vi "ATC예문.vi"() -> ()   [LabVIEW 2014]
doc: "ATC app"
uses:
  <vilib>/Utility/sysdir.llb/System Directory Type.ctl
panel:
  in  "피드백":bool
  in  "정보1":bool
  in  "도움말":bool
  in  "정규식 5":string
  in  "정규식 4":string
  in  "?":bool
  in  "?":bool
  in  "정규식 3":string
  out "ip address":string="ip address"
  in  "탭":T1(tab)
  in  "메모":string="필요한 메모를 할수 있습니다. "
  in  "SID&RadarVector. 2":string="SID&RadarVector. "
  in  "인사말":string="인사말"
  in  "CD관제기관":string="관제기관"
  in  "콜사인":string="콜사인\n콜사인\n콜사인"
  in  "도착공항":string="도착공항"
  in  "SID&RadarVector":string="SID&RadarVector"
  in  "비행고도":string="비행고도"
  in  "인사말2":string="인사말"
  in  "콜사인2":string="콜사인"
  in  "콜사인3":string="콜사인"
  in  "콜사인4":string="콜사인"
  in  "콜사인5":string="콜사인"
  in  "콜사인6":string="콜사인"
  in  "도착공항2":string="도착공항"
  in  "제한고도":string="제한고도"
  in  "비행고도2":string="비행고도"
  in  "D접속주파수":string="접속주파수"
  in  "스콱번호":string="스콱번호"
  in  "도착공항3":string="도착공항"
  in  "SID&RadarVector. 3":string="SID&RadarVector. "
  in  "제한고도2":string="제한고도"
  in  "비행고도3":string="비행고도"
  in  "D접속주파수2":string="접속주파수"
  in  "스콱번호2":string="스쾃번호"
  in  "콜사인7":string="콜사인"
  in  "콜사인8":string="콜사인"
  in  "G관제기관":string="관제기관"
  in  "G접속주파수2":string="접속주파수"
  in  "G관제기관2":string="관제기관"
  in  "G접속주파수":string="접속주파수"
  in  "콜사인9":string="콜사인"
  in  "유도로 2":string="유도로"
  in  "유도로":string="유도로"
  in  "방향 2":string="방향"
  in  "방향":string="방향"
  in  "메모2":string="필요한 메모를 할수 있습니다. "
  in  "T관제기관2":string="관제기관"
  in  "콜사인24":string="콜사인"
  in  "T접속주파수2":string="접속주파수"
  in  "T접속주파수":string="접속주파수"
  in  "T관제기관":string="관제기관"
  in  "콜사인23":string="콜사인"
  in  "활주로9":string="활주로"
  in  "G관제기관4":string="관제기관"
  in  "콜사인22":string="콜사인"
  in  "콜사인21":string="콜사인"
  in  "콜사인20":string="콜사인"
  in  "콜사인19":string="콜사인"
  in  "활주로8":string="활주로"
  in  "활주로7":string="활주로"
  in  "콜사인17":string="콜사인"
  in  "활주로6":string="활주로"
  in  "콜사인18":string="콜사인"
  in  "활주로5":string="활주로"
  in  "콜사인16":string="콜사인"
  in  "활주로4":string="활주로"
  in  "콜사인15":string="콜사인"
  in  "활주로3":string="활주로"
  in  "콜사인14":string="콜사인"
  in  "콜사인13":string="콜사인"
  in  "현재기압2":string="현재기압"
  in  "출발공항":string="출발공항"
  in  "활주로2":string="활주로"
  in  "현재기압":string="현재기압"
  in  "출발공항2":string="출발공항"
  in  "활주로1":string="활주로"
  in  "콜사인12":string="콜사인"
  in  "콜사인11":string="콜사인"
  in  "G관제기관3":string="관제기관"
  in  "인사3":string="인사"
  in  "콜사인34 2":string="콜사인"
  in  "D관제기관2":string="관제기관"
  in  "D관제기관":string="관제기관"
  in  "T관제기관3":string="관제기관"
  in  "메모3":string="필요한 메모를 할수 있습니다. "
  in  "인사4":string="인사"
  in  "콜사인25":string="콜사인"
  in  "활주로10":string="활주로"
  in  "콜사인26":string="콜사인"
  in  "바람방향":string="바람방향"
  in  "풍속":string="풍속"
  in  "콜사인28":string="콜사인"
  in  "활주로13":string="활주로"
  in  "콜사인29":string="콜사인"
  in  "활주로12":string="활주로"
  in  "콜사인30":string="콜사인"
  in  "활주로14":string="활주로"
  in  "콜사인31":string="콜사인"
  in  "활주로15":string="활주로"
  in  "T관제기관4":string="관제기관"
  in  "콜사인32":string="콜사인"
  in  "현재고도":string="현재고도"
  in  "허가고도":string="허가고도"
  in  "콜사인33":string="콜사인"
  in  "접속주파수":string="접속주파수"
  in  "콜사인34":string="콜사인"
  in  "접속주파수2":string="접속주파수"
  in  "순항고도or이니셜고도":string="순항고도or이니셜고도"
  in  "D관제기관5":string="관제기관"
  in  "메모 4":string="필요한 메모를 할수 있습니다. "
  in  "인사5":string="인사"
  in  "D관제기관3":string="관제기관"
  in  "콜사인35":string="콜사인"
  in  "현재고도A":string="현재고도"
  in  "콜사인36":string="콜사인"
  in  "D관제기관4":string="관제기관"
  in  "허가고도4":string="허가고도"
  in  "허가고도5":string="허가고도"
  in  "콜사인37":string="콜사인"
  in  "콜사인38":string="콜사인"
  in  "허가고도6":string="허가고도"
  in  "허가고도7":string="허가고도"
  in  "콜사인39":string="콜사인"
  in  "콜사인40":string="콜사인"
  in  "C관제기관":string="관제기관"
  in  "A접속주파수":string="접속주파수"
  in  "C관제기관2":string="관제기관"
  in  "A접속주파수2":string="접속주파수"
  in  "콜사인41":string="콜사인"
  in  "콜사인38 2":string="콜사인"
  in  "D관제기관6":string="관제기관"
  in  "허가고도6 2":string="허가고도"
  in  "허가고도6 3":string="허가고도"
  in  "콜사인39 2":string="콜사인"
  in  "메모5":string="필요한 메모를 할수 있습니다. "
  in  "인사말 2":string="인사말"
  in  "허가고도 2":string="허가고도"
  in  "지점":string="지점"
  in  "허가고도7 2":string="허가고도"
  in  "콜사인38 3":string="콜사인"
  in  "콜사인39 3":string="콜사인"
  in  "허가고도7 3":string="허가고도"
  in  "지점 2":string="지점"
  in  "메모6":string="필요한 메모를 할수 있습니다. "
  in  "A관제기관3":string="관제기관"
  in  "콜사인46":string="콜사인"
  in  "날시정보":string="날시정보"
  in  "고도":string="고도"
  in  "콜사인47":string="콜사인"
  in  "A관제기관4":string="관제기관"
  in  "L활주로":string="활주로"
  in  "도착공항4":string="도착공항"
  in  "현재기압":string="현재기압"
  in  "콜사인48":string="콜사인"
  in  "A관제기관5":string="관제기관"
  in  "L활주로":string="활주로"
  in  "도착공항5":string="도착공항"
  in  "현재기압":string="현재기압"
  in  "콜사인49":string="콜사인"
  in  "고도":string="고도"
  in  "콜사인50":string="콜사인"
  in  "고도":string="고도"
  in  "콜사인51":string="콜사인"
  in  "고도":string="고도"
  in  "고도":string="고도"
  in  "콜사인52":string="콜사인"
  in  "콜사인53":string="콜사인"
  in  "A관제기관":string="관제기관"
  in  "풍속":string="풍속"
  in  "바람방향":string="바람방향"
  in  "L활주로3":string="활주로"
  in  "콜사인54":string="콜사인"
  in  "L활주로":string="활주로"
  in  "콜사인55":string="콜사인"
  in  "A관제기관2":string="관제기관"
  in  "L활주로":string="활주로"
  in  "ILS":string="주파수(ils)"
  in  "콜사인56":string="콜사인"
  in  "L활주로6":string="활주로"
  in  "ILS2":string="주파수(ils)"
  in  "콜사인57":string="콜사인"
  in  "T관제기관":string="관제기관"
  in  "T접속주파수":string="접속주파수"
  in  "콜사인58":string="콜사인"
  in  "콜사인59":string="콜사인"
  in  "관제기관":string="관제기관"
  in  "T접속주파수":string="접속주파수"
  in  "메모7":string="필요한 메모를 할수 있습니다. "
  in  "바람방향":string="바람방향"
  in  "관제기관":string="관제기관"
  in  "콜사인60":string="콜사인"
  in  "L활주로7":string="활주로"
  in  "콜사인61":string="콜사인"
  in  "풍속":string="풍속"
  in  "콜사인62":string="콜사인"
  in  "L활주로":string="활주로"
  in  "L활주로":string="활주로"
  in  "관제기관":string="관제기관"
  in  "콜사인63":string="콜사인"
  in  "관제기관3":string="관제기관"
  in  "콜사인64":string="콜사인"
  in  "L활주로":string="활주로"
  in  "G관제기관":string="관제기관"
  in  "G접속주파수":string="접속주파수"
  in  "콜사인65":string="콜사인"
  in  "관제기관":string="관제기관"
  in  "G접속주파수":string="접속주파수"
  in  "콜사인70":string="콜사인"
  in  "C활주로3":string="활주로"
  in  "C활주로2":string="활주로"
  in  "관제기관3 2":string="관제기관"
  in  "C활주로":string="활주로"
  in  "콜사인69":string="콜사인"
  in  "관제기관2":string="관제기관"
  in  "메모8":string="필요한 메모를 할수 있습니다. "
  in  "관제기관":string="관제기관"
  in  "콜사인66":string="콜사인"
  in  "콜사인67":string="콜사인"
  in  "게이트번호":string="게이트번호"
  in  "THEN":string="then"
  in  "콜사인68":string="콜사인"
  in  "게이트번호2":string="게이트번호"
  in  "THEN2":string="then"
  in  "콜사인10":string="콜사인"
  in  "관제기관4":string="관제기관"
  in  "콜사인71":string="콜사인"
  in  "콜사인72":string="콜사인"
  # "ver.3.0.0.55"
  # "~"
  # "Good"
  # "Clearance Delivery"
  # "Pilot"
  # "at FL"
  # "Request IFR Clearance to"
  # "Airport via"
  # "~"
  # "Good"
  # "Controller"
  # ",  Clearance  Delivery, standby."
  # "Pilot"
  # "Stand by,"
  # "Controller"
  # "Delivery 또는 Delivery, Are you ready to copy?"
  # "Pilot"
  # "Go Ahead 또는 Ready to copy"
  # "Airport via"
  # ", Cleared to"
  # "Controller"
  # "ft expect FL"
  # "then as filed. Climb and Maintain"
  # "Departure Frequency"
  # "Read back."
  # "Squawk"
  # "Pilot"
  # "Airport via"
  # "Cleared to"
  # ","
  # "then as filed."
  # "Climb and Maintain"
  # "ft expect FL"
  # "Departure Frequency"
  # "and  Squawk"
  # "Controller"
  # ", Read back is corrent contact"
  # "Ground"
  # "bye bye~."
  # "Pilot"
  # "Roger, contact"
  # ", bye bye~"
  # "Pilot"
  # "Good"
  # "~"
  # "ready for push back and Engine Start."
  # ","
  # ", Rwy"
  # "Push Back and Engine Start Approved, heading to"
  # "Controller"
  # ","
  # "QNH"
  # "Read Back."
  # "Pilot"
  # "Roger\nPush Back and Engine Start Approved, heading to"
  # ", Rwy"
  # "QNH"
  # "Ready for taxi to the Rwy"
  # ","
  # "Pilot"
  # "- Push back 완료 후 -"
  # ", Ready for Taxi to Rwy"
  # "Controller"
  # ", taxi to"
  # "via taxiway"
  # ", Roger"
  # "Pilot"
  # "via taxiway"
  # "Taxi to"
  # "- 활주로를 건널 상황일 때 -"
  # "Pilot"
  # "Request Cross Rwy"
  # "Controller"
  # ", cleared Cross Rwy"
  # "Pilot"
  # "cleared Cross Rwy"
  # "Controller"
  # "Squawk Mode C."
  # "Pilot"
  # ", Roger squawk mode 'C'"
  # "------------------------ 홀딩 포인트 도착 후 ----------------------------------"
  # "Pilot"
  # "hold short of Rwy"
  # ","
  # "Controller"
  # "Roger,"
  # "contact"
  # "Tower"
  # "bye bye~"
  # "Pilot"
  # "Contact"
  # "Pilot"
  # "Good"
  # "~"
  # ",  hold short Rwy"
  # ", Ready for Departure"
  # "(곧바로 이륙허가)"
  # "Controller"
  # ", wind"
  # "knot, cleared for take off."
  # "at"
  # "(활주로 정렬대기)"
  # "Controller"
  # "Line up and wait Rwy"
  # "Pilot"
  # "Line up and wait Rwy"
  # "Roger,"
  # "(홀딩 포인트에서 대기)"
  # "Controller"
  # ", Hold short rwy"
  # ","
  # "Pilot"
  # "Hold short of Rwy"
  # "Roger,"
  # "- 이 륙 후 -"
  # "Pilot"
  # "ft."
  # "Airborn Passing"
  # "ft, Climbing"
  # ","
  # "Controller"
  # ", contact"
  # "Departure,"
  # "bye bye~"
  # "Pilot"
  # ", Roger"
  # "Contact"
  # "Departure,"
  # "bye bye~"
  # "Good"
  # "~"
  # "Pilot"
  # "Passing"
  # "expect"
  # "with (SID)."
  # ","
  # ","
  # "Controller"
  # "Departure, Radar Contact, Climb via (SID) to"
  # ","
  # "."
  # "Pilot"
  # "Roger, Climb via"
  # ","
  # "-고도제한 해제시-"
  # "Controller"
  # "Departure, Radar Contact, Climb via (SID) to"
  # ", Cancel Level Restrictions."
  # "Pilot"
  # "Roger, Climb via (SID) to"
  # ", Cancel Level Restrictions,"
  # "-속도제한 해제시-"
  # "Controller"
  # "Departure, Radar Contact, Climb via (SID) to"
  # ", Cancel Speed Restrictions."
  # "Pilot"
  # "Roger, Climb via (SID) to"
  # ", Cancel Speed Restrictions,"
  # "Controller"
  # "Control,"
  # ", bye bye."
  # ", You are leaving my airspace, Contact"
  # "Pilot"
  # "Contact"
  # "G'day"
  # "Control,"
  # ","
  # "Pilot"
  # "Good"
  # "Decend and maintain FL"
  # "with (SID)."
  # "-하강 발부-"
  # "Controller"
  # "by"
  # ", Descend and Maintain"
  # "Pilot"
  # "Descend and Maintain"
  # "by"
  # "Pilot"
  # ","
  # "FL"
  # "with information"
  # ","
  # ", Expect vector to ILS Rwy"
  # "approach"
  # "Controller"
  # "QNH"
  # "Roger,"
  # "Pilot"
  # ", Expect vector to ILS Rwy"
  # "final approach"
  # "QNH"
  # "Controller"
  # ", Decend and maintain FL"
  # "Pilot"
  # "Decend and maintain FL"
  # "Roger,"
  # "Controller"
  # ", Decend and maintain"
  # "ft"
  # "Pilot"
  # "Roger"
  # "Decend and maintain"
  # "ft"
  # "Controller"
  # ","
  # "for landing"
  # "wind"
  # "knots active Rwy"
  # "at"
  # "Pilot"
  # "Roger,"
  # "Rwy"
  # "for landing"
  # "Controller"
  # ","
  # "approach use Rwy"
  # "ILS"
  # "Roger,"
  # "Pilot"
  # "Use Rwy"
  # "ILS"
  # "- 정 렬 후 -"
  # "Pilot"
  # "Approach,"
  # ", Established on Localizer."
  # "Controller"
  # "Tower,"
  # "Good day,"
  # "Roger, Contact"
  # "Pilot"
  # "Contact"
  # "Tower"
  # "Good day,"
  # "Pilot"
  # ","
  # "Inbound Approaching Rwy"
  # "Controller"
  # ", Wind"
  # "at"
  # "knots Rwy"
  # ", Cleared to land"
  # "Pilot"
  # "Rwy"
  # "Cleared to land"
  # "Pilot"
  # ","
  # "- 착 륙 후 -"
  # ","
  # "Pilot"
  # "Touch down with Rwy"
  # "Controller"
  # "Roger, change squawk mode Standby and contact"
  # "bye bye~"
  # "ground"
  # "Pilot"
  # ", Roger"
  # "bye bye~"
  # "Change squawk mode standby and contact"
  # "- 활주로를 건널 상황일 때 -"
  # "Pilot"
  # ","
  # "Request Cross Rwy"
  # "Controller"
  # ", Cross Rwy"
  # "approved."
  # "Pilot"
  # "Cross Rwy"
  # "approved"
  # ","
  # "Pilot"
  # "Ready to taxi to the Gate"
  # "Controller"
  # ", taxi to the gate"
  # "via taxi way"
  # "Roger,"
  # "Pilot"
  # "taxi to the gate"
  # "via taxi way"
  # "- 게이트 도착 후 -"
  # "Pilot"
  # "at Gate and Engine Shut down."
  # "Thank you for your ATC service."
  # "Controller"
  # ", at the gate and Engine Shut down, Thank you ~~"
  # "Pilot"
  # "Have a nice day,"
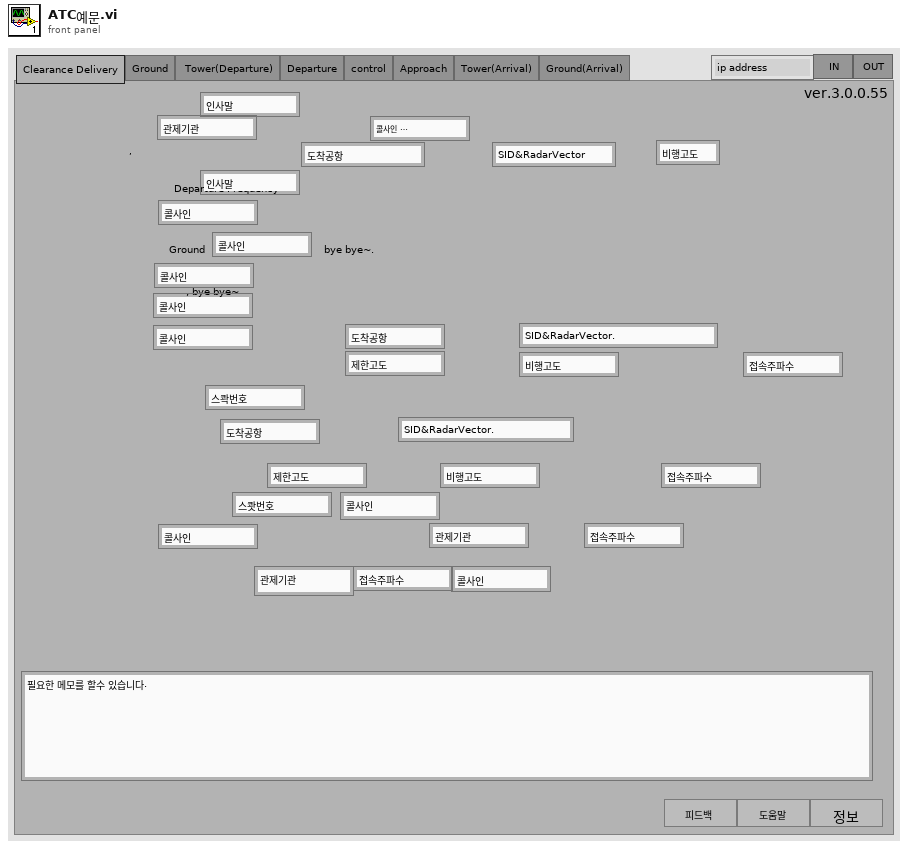
[diagram p1: front panel]
types:
  T1 = enum32{"Clearance Delivery", "Ground", " Tower(Departure)", "Departure", "control", "Approach", "Tower(Arrival)", "Ground(Arrival)"}
  T2 = enum16{"open", "replace", "create", "open or create", "replace or create", "replace or create with confirmation"}
  T3 = typedef "System Directory Type.ctl" = i32
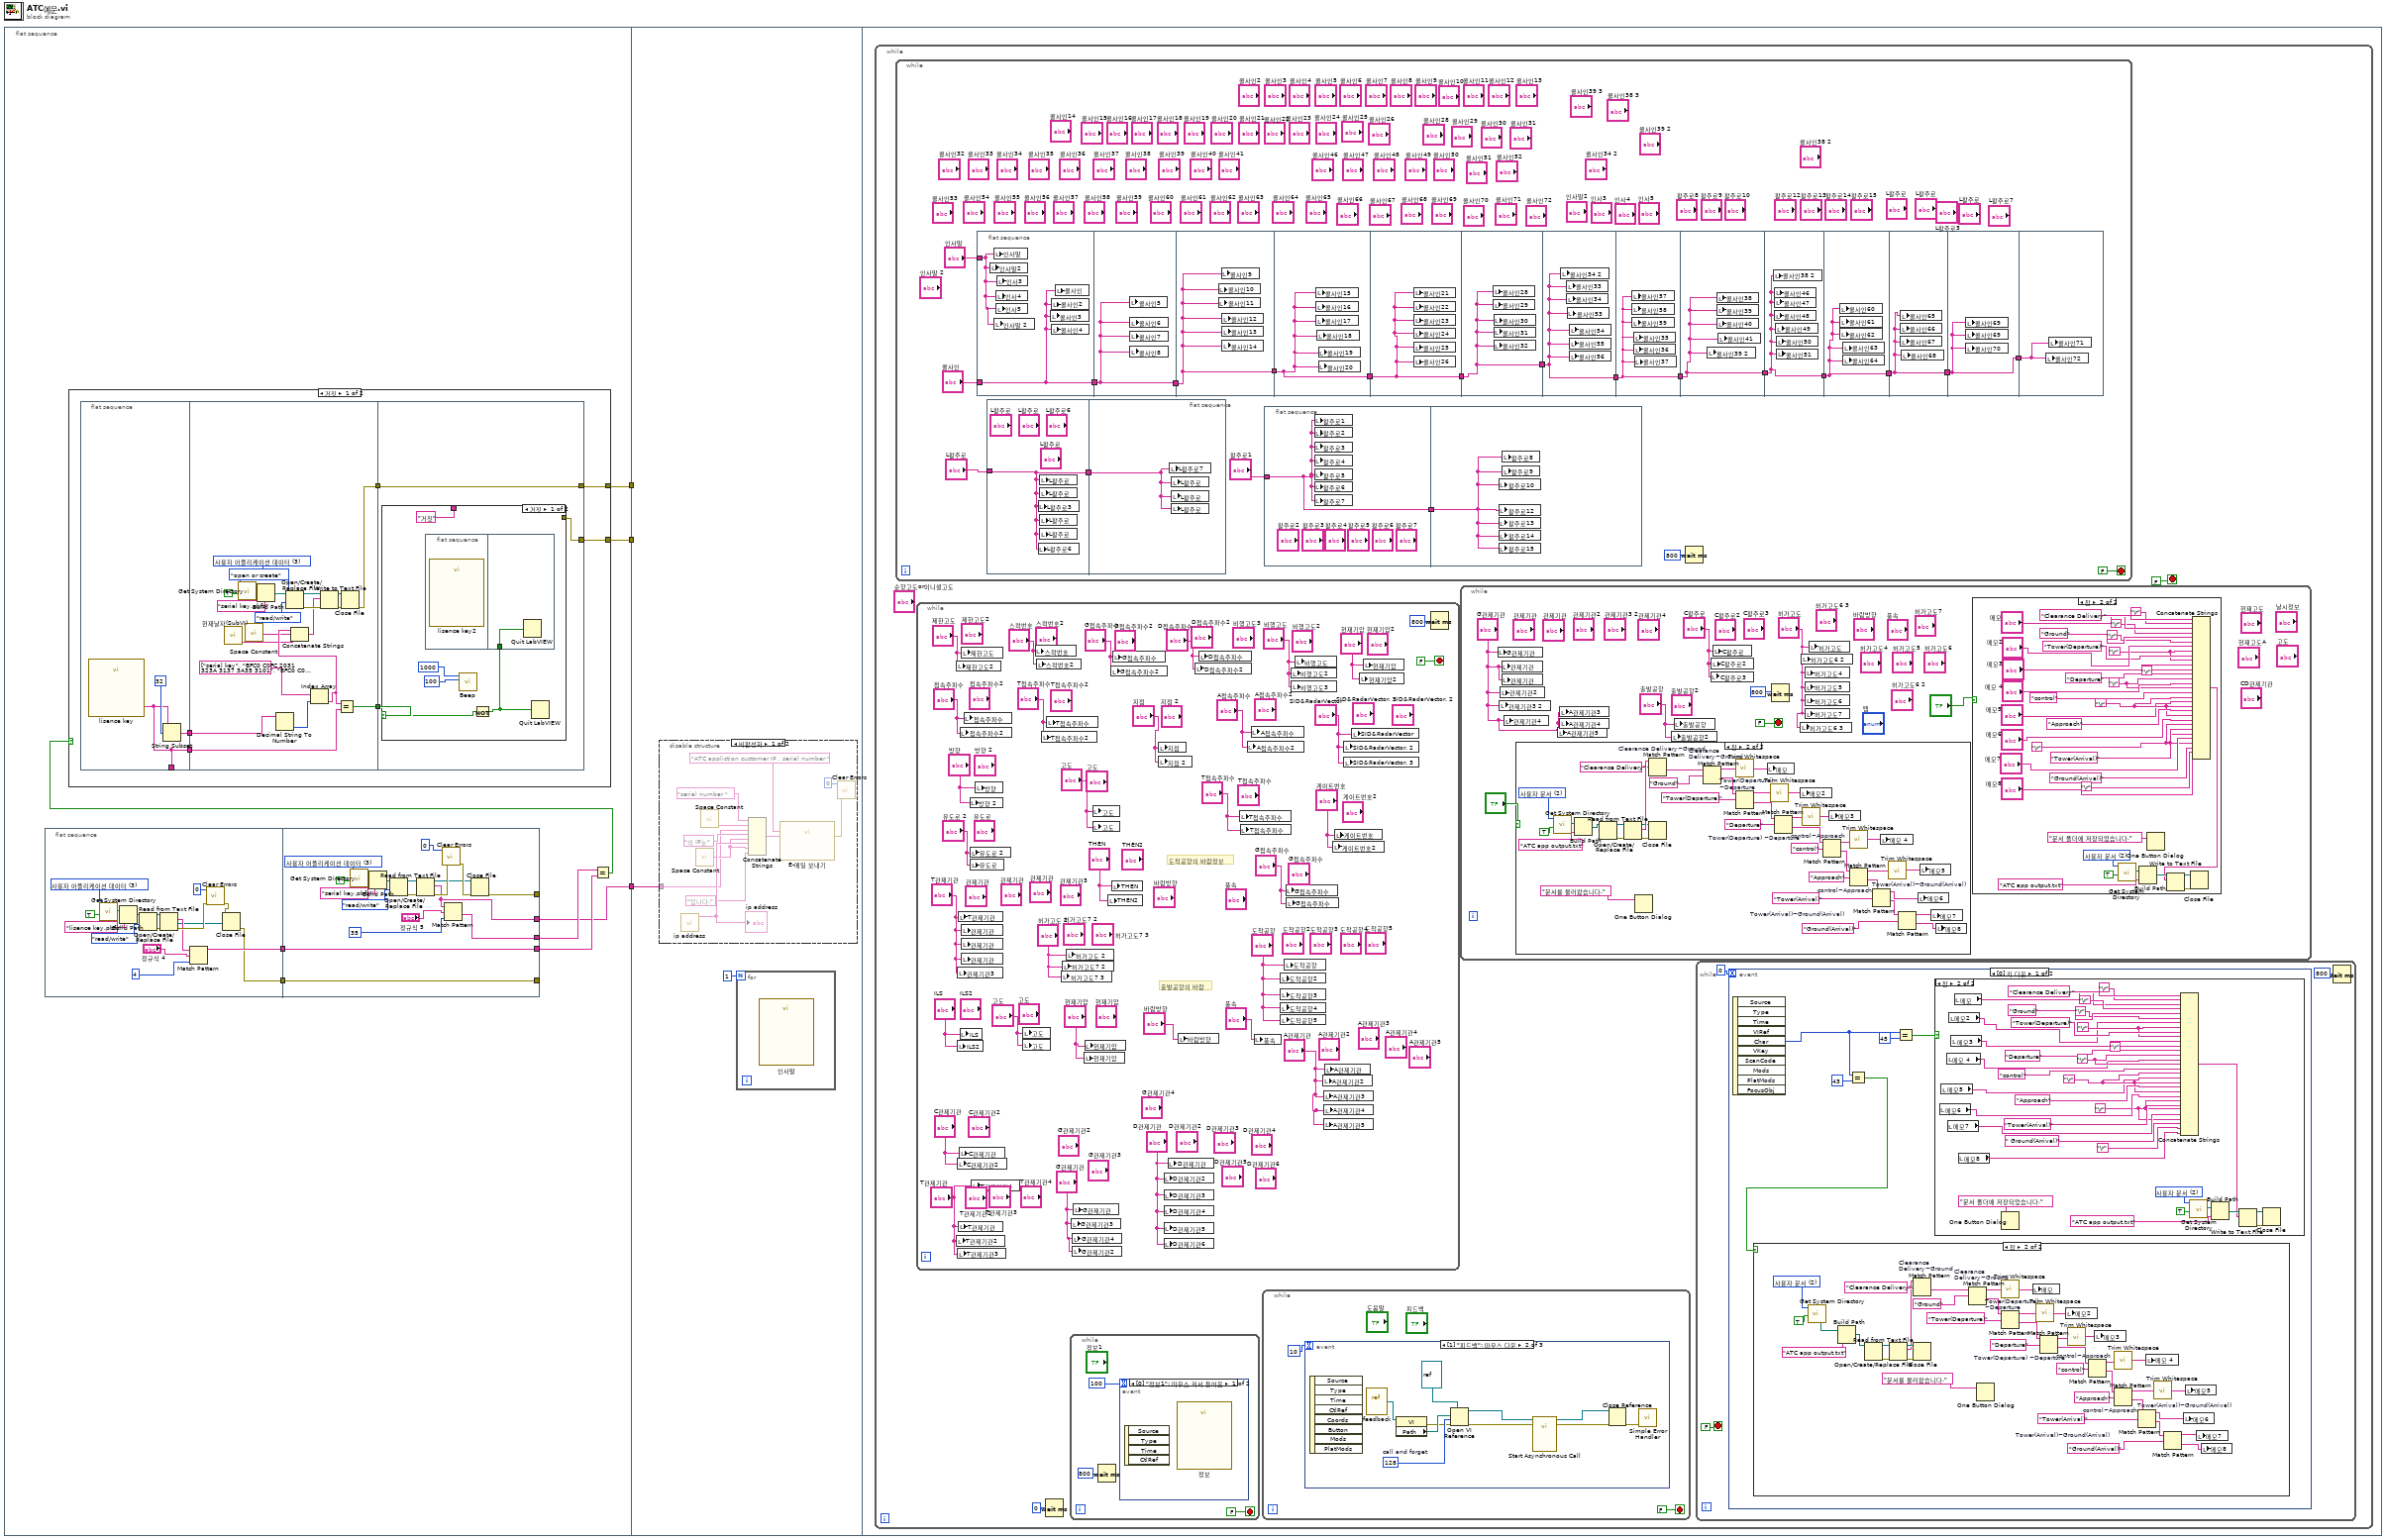
[diagram p0: block diagram]
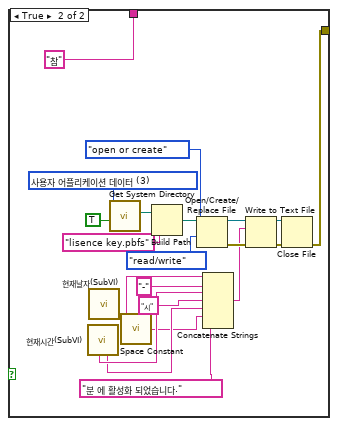
[diagram p2: hidden frame]
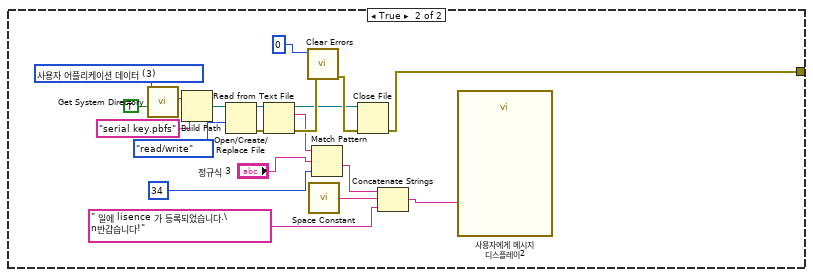
[diagram p3: hidden frame]
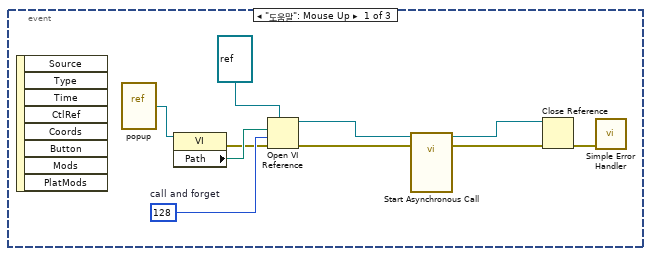
[diagram p5: hidden frame]
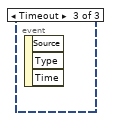
[diagram p6: hidden frame]
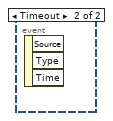
[diagram p9: hidden frame]
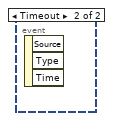
[diagram p10: hidden frame]
diagram:
  n1 = flat-sequence {
    tunnel: [w4] -> w3
    tunnel: [w11] -> w2
    tunnel: [w10] -> w1
    tunnel: w3 -> [w128]
    tunnel: w2 -> [_]
    tunnel: w1 -> [_]
    frame #0 {
      n2 = flat-sequence {
        tunnel: [w13] -> w9
        tunnel: [w12] -> w8
        tunnel: [w35] -> w6
        tunnel: w9 -> [w35]
        tunnel: [w33] -> w7
        tunnel: [w29] -> w4
        tunnel: [w31] -> _
        tunnel: w8 -> [w31]
        tunnel: [w30] -> _
        frame #0 {
          w18 = T3 3 items=["사용자 홈"=0, "사용자 데스크탑"=1, "사용자 문서"=2, "사용자 어플리케이션 데이터"=3, "사용자 환경"=4, "사용자 임시"=5, "퍼블릭 문서"=6, "퍼블릭 어플리케이션 데이터"=7, "퍼블릭 환경"=8, "퍼블릭 캐시"=13, "시스템 코어 라이브러리"=9, "시스템 설치된 라이브러리"=10, "어플리케이션 파일"=11, "부팅 볼륨 루트"=12] ("system directory type")
          n3 = call <vilib>:"Get System Directory.vi"("create directory if not found? (F)"=TRUE, "system directory type"=w18) -> ("system directory"=w17:path)  [unwired: 9 in]
          n4 = Build Path(base path=w17, name or relative path="lisence key.pbfs" ("이름 또는 상대 경로")) -> (appended path=w16:path)
          n5 = Open/Create/Replace File(file path (use dialog)=w16, access (0:read/write)=enum16{"read/write", "read-only", "write-only"}."read/write" ("접근(0:읽기/쓰기)")) -> (refnum out=w22:refnum<file>, error out=w21:errorcluster)  [unwired: 4 in, 1 out]
          n6 = Read from Text File(file (use dialog)=w22, error in=w21) -> (refnum out=w23:refnum<file>, text=w24:string, error out=w26:errorcluster)  [unwired: 2 in, 1 out]
          n7 = Match Pattern(string=w24, regular expression="정규식 4", offset (0)=4 ("오프셋(0) 2")) -> (before substring=w13:string)  [unwired: 3 out]
          n8 = call <vilib>:"Clear Errors.vi"("error in (no error)"=w26, "specific error code to clear (0: all)"=0) -> ("error out"=w27:errorcluster)  [unwired: 4 in, 1 out]
          n9 = Close File(refnum=w23, error in=w27) -> (error out=w12:errorcluster)  [unwired: 1 out]
        }
        frame #1 {
          w41 = T3 3 items=["사용자 홈"=0, "사용자 데스크탑"=1, "사용자 문서"=2, "사용자 어플리케이션 데이터"=3, "사용자 환경"=4, "사용자 임시"=5, "퍼블릭 문서"=6, "퍼블릭 어플리케이션 데이터"=7, "퍼블릭 환경"=8, "퍼블릭 캐시"=13, "시스템 코어 라이브러리"=9, "시스템 설치된 라이브러리"=10, "어플리케이션 파일"=11, "부팅 볼륨 루트"=12] ("system directory type")
          n10 = call <vilib>:"Get System Directory.vi"("create directory if not found? (F)"=TRUE, "system directory type"=w41) -> ("system directory"=w42:path)  [unwired: 9 in]
          n11 = Build Path(base path=w42, name or relative path="serial key.pbfs" ("이름 또는 상대 경로")) -> (appended path=w43:path)
          n12 = Open/Create/Replace File(file path (use dialog)=w43, access (0:read/write)=enum16{"read/write", "read-only", "write-only"}."read/write" ("접근(0:읽기/쓰기)")) -> (refnum out=w37:refnum<file>, error out=w38:errorcluster)  [unwired: 4 in, 1 out]
          n13 = Read from Text File(file (use dialog)=w37, error in=w38) -> (refnum out=w36:refnum<file>, text=w29:string, error out=w45:errorcluster)  [unwired: 2 in, 1 out]
          n14 = call <vilib>:"Clear Errors.vi"("error in (no error)"=w45, "specific error code to clear (0: all)"=0) -> ("error out"=w46:errorcluster)  [unwired: 4 in, 1 out]
          n15 = Match Pattern(string=w29, regular expression="정규식 5", offset (0)=35 ("오프셋(0)")) -> (after substring=w33:string)  [unwired: 3 out]
          n16 = Close File(refnum=w36, error in=w46) -> (error out=w30:errorcluster)  [unwired: 1 out]
        }
      }
      n17 = Equal?(x=w7, y=w6) -> (x = y?=w5:bool)
      n18 = case shown="거짓" w5 {
        tunnel: [w49 w108] -> w10
        tunnel: [w48 _] -> w11
        frame False {
          n19 = flat-sequence {
            tunnel: [w55] -> w53
            tunnel: [w54] -> w52
            tunnel: [w54] -> _
            tunnel: w53 -> [w77]
            tunnel: [w74] -> w51
            tunnel: w52 -> [w75]
            tunnel: [w58] -> w50
            tunnel: w51 -> [w80]
            tunnel: [w79] -> w49
            tunnel: w50 -> [w78]
            tunnel: [w78] -> w48
            frame #0 {
              n20 = call "lisence key"() -> ("lisence key"=w54:string)  [unwired: 17 in, 2 out]
              n21 = String Subset(string=w54, offset (0)=32 ("오프셋(0)")) -> (substring=w55:string)  [unwired: 1 in]
            }
            frame #1 {
              w67 = T3 3 items=["사용자 홈"=0, "사용자 데스크탑"=1, "사용자 문서"=2, "사용자 어플리케이션 데이터"=3, "사용자 환경"=4, "사용자 임시"=5, "퍼블릭 문서"=6, "퍼블릭 어플리케이션 데이터"=7, "퍼블릭 환경"=8, "퍼블릭 캐시"=13, "시스템 코어 라이브러리"=9, "시스템 설치된 라이브러리"=10, "어플리케이션 파일"=11, "부팅 볼륨 루트"=12] ("system directory type")
              n22 = call "현재날자(SubVI).vi"() -> ("월,일 을 문자열로"=w62:string)  [unwired: 5 in, 6 out]
              n23 = call <vilib>:"Get System Directory.vi"("create directory if not found? (F)"=TRUE, "system directory type"=w67) -> ("system directory"=w66:path)  [unwired: 9 in]
              n24 = call <vilib>:"Space Constant.vi"() -> ("String"=w61:string)
              n25 = Build Path(base path=w66, name or relative path="serial key.pbfs" ("이름 또는 상대 경로")) -> (appended path=w65:path)
              n26 = Decimal String To Number(string=w77) -> (number=w76:i32)  [unwired: 2 in, 1 out]
              n27 = Open/Create/Replace File(file path (use dialog)=w65, operation (0:open)=T2."open or create" ("동작(0:open)"), access (0:read/write)=enum16{"read/write", "read-only", "write-only"}."read/write" ("접근(0:읽기/쓰기)")) -> (refnum out=w73:refnum<file>, error out=w72:errorcluster)  [unwired: 3 in, 1 out]
              n28 = Index Array(array=string[] ["serial key", "BFC0 C0FC 2031 323A 3137 3A35 3101", "BFC0 C0FC 2031 323A 3138 3A30 3902", "BFC0 C0FC 2031 323A 3139 3A30 3903", "BFC0 C0FC 2031 323A 3230 3A30 3904", "BFC0 C0FC 2031 323A 3231 3A30 3905", "BFC0 C0FC 2031 323A 3232 3A30 3906", "BFC0 C0FC 2031 323A 3233 3A30 3907", "BFC0 C0FC 2031 323A 3234 3A30 3908", "BFC0 C0FC 2031 323A 3235 3A30 3909", "BFC0 C0FC 2031 323A 3236 3A30 3910", "BFC0 C0FC 2031 323A 3237 3A30 3911", "BFC0 C0FC 2031 323A 3238 3A30 3912", "BFC0 C0FC 2031 323A 3239 3A30 3913", "BFC0 C0FC 2031 323A 3036 3A33 3214", "BFC0 C0FC 2031 323A 3037 3A33 3215", "BFC0 C0FC 2031 323A 3038 3A33 3216", "BFC0 C0FC 2031 323A 3038 3A33 3217", "BFC0 C0FC 2031 323A 3039 3A33 3218", "BFC0 C0FC 2031 323A 3039 3A35 3019", "BFC0 C0FC 2031 323A 3130 3A35 3020", "BFC0 C0FC 2031 323A 3131 3A35 3121", "BFC0 C8C4 2031 313A 3536 3A33 3222", "BFC0 C8C4 2031 313A 3537 3A33 3223", "BFC0 C8C4 2031 313A 3538 3A33 3224", "BFC0 C8C4 2031 313A 3539 3A33 3225", "BFC0 C0FC 2031 323A 3030 3A33 3226", "BFC0 C0FC 2031 323A 3031 3A33 3227", "BFC0 C0FC 2031 323A 3032 3A33 3228", "BFC0 C0FC 2031 323A 3033 3A33 3229", "BFC0 C0FC 2031 323A 3034 3A33 3230", "BFC0 C0FC 2031 323A 3035 3A33 3231", "BFC0 C0FC 2031 323A 3036 3A33 3232", "BFC0 C0FC 2031 323A 3037 3A33 3233", "BFC0 C0FC 2031 323A 3038 3A33 3234", "BFC0 C0FC 2033 3A34 373A 3031 0035 ", "BFC0 C0FC 2033 3A34 383A 3234 0036", "BFC0 C0FC 2033 3A34 393A 3132 0037", "BFC0 C0FC 2033 3A35 303A 3534 0038", "BFC0 C0FC 2033 3A35 313A 3231 0039 ", "BFC0 C0FC 2033 3A35 323A 3333 0040 ", "BFC0 C0FC 2033 3A35 333A 3030 0041", "BFC0 C0FC 2033 3A35 343A 3432 0042", "BFC0 C0FC 2033 3A35 353A 3431 0043", "BFC0 C0FC 2033 3A35 363A 3131 0044", "BFC0 C0FC 2033 3A35 373A 3239 0045", "BFC0 C0FC 2033 3A35 383A 3539 0046", "BFC0 C0FC 2033 3A35 393A 3533 0047", "BFC0 C0FC 2034 3A30 303A 3430 0048 "] ("출력 배열"), index=w76) -> (element=w63:string)
              n29 = Concatenate Strings(w63, w61, w62) -> (w64:string)
              n30 = Write to Text File(file (use dialog)=w73, text=w64, error in=w72) -> (refnum out=w70:refnum<file>, error out=w71:errorcluster)  [unwired: 1 in, 1 out]
              n31 = Equal?(x=w63, y=w75) -> (x = y?=w74:bool)
              n32 = Close File(refnum=w70, error in=w71) -> (error out=w58:errorcluster)  [unwired: 1 out]
            }
            frame #2 {
              n33 = case shown="거짓" w80 {
                selector: w80 -> [w83 _]
                tunnel: ["거짓" "참"] -> _
                tunnel: [_ w87] -> w79
                frame False {
                  n34 = flat-sequence {
                    tunnel: w84 -> [w86]
                    frame #0 {
                      n35 = call "lisence key2"() -> ()  [unwired: 10 in, 2 out]
                    }
                    frame #1 {
                      n36 = Quit LabVIEW(quit? (T)=w86) -> ()
                    }
                  }
                  n37 = call <vilib>:"Beep.vi"("duration (msec)"=u32 100, "frequency (Hz)"=u32 1000) -> ()  [unwired: 10 in]
                  n38 = Not(x=w83) -> (.not. x?=w84:bool)
                  n39 = Quit LabVIEW(quit? (T)=w84) -> ()
                }
                frame True {
                  w103 = T3 3 items=["사용자 홈"=0, "사용자 데스크탑"=1, "사용자 문서"=2, "사용자 어플리케이션 데이터"=3, "사용자 환경"=4, "사용자 임시"=5, "퍼블릭 문서"=6, "퍼블릭 어플리케이션 데이터"=7, "퍼블릭 환경"=8, "퍼블릭 캐시"=13, "시스템 코어 라이브러리"=9, "시스템 설치된 라이브러리"=10, "어플리케이션 파일"=11, "부팅 볼륨 루트"=12] ("system directory type")
                  n40 = call "현재시간(SubVI).vi"() -> ("분 문자열"=w92:string, "시 문자열"=w94:string)  [unwired: 3 in, 7 out]
                  n41 = call "현재날자(SubVI).vi"() -> ("월,일 을 문자열로"=w96:string)  [unwired: 5 in, 6 out]
                  n42 = call <vilib>:"Get System Directory.vi"("create directory if not found? (F)"=TRUE, "system directory type"=w103) -> ("system directory"=w104:path)  [unwired: 9 in]
                  n43 = call <vilib>:"Space Constant.vi"() -> ("String"=w91:string)
                  n44 = Build Path(base path=w104, name or relative path="lisence key.pbfs" ("이름 또는 상대 경로")) -> (appended path=w105:path)
                  n45 = Open/Create/Replace File(file path (use dialog)=w105, operation (0:open)=T2."open or create" ("동작(0:open)"), access (0:read/write)=enum16{"read/write", "read-only", "write-only"}."read/write" ("접근(0:읽기/쓰기)")) -> (refnum out=w101:refnum<file>, error out=w99:errorcluster)  [unwired: 3 in, 1 out]
                  n46 = Concatenate Strings(w96, "-", w94, "시", w92, w91, "분 에 활성화 되었습니다.") -> (w97:string)
                  n47 = Write to Text File(file (use dialog)=w101, text=w97, error in=w99) -> (refnum out=w102:refnum<file>, error out=w98:errorcluster)  [unwired: 1 in, 1 out]
                  n48 = Close File(refnum=w102, error in=w98) -> (error out=w87:errorcluster)  [unwired: 1 out]
                }
              }
            }
          }
        }
        frame True {
          w121 = T3 3 items=["사용자 홈"=0, "사용자 데스크탑"=1, "사용자 문서"=2, "사용자 어플리케이션 데이터"=3, "사용자 환경"=4, "사용자 임시"=5, "퍼블릭 문서"=6, "퍼블릭 어플리케이션 데이터"=7, "퍼블릭 환경"=8, "퍼블릭 캐시"=13, "시스템 코어 라이브러리"=9, "시스템 설치된 라이브러리"=10, "어플리케이션 파일"=11, "부팅 볼륨 루트"=12] ("system directory type")
          n49 = call <vilib>:"Get System Directory.vi"("create directory if not found? (F)"=TRUE, "system directory type"=w121) -> ("system directory"=w122:path)  [unwired: 9 in]
          n50 = Build Path(base path=w122, name or relative path="serial key.pbfs" ("이름 또는 상대 경로")) -> (appended path=w123:path)
          n51 = Open/Create/Replace File(file path (use dialog)=w123, access (0:read/write)=enum16{"read/write", "read-only", "write-only"}."read/write" ("접근(0:읽기/쓰기)")) -> (refnum out=w117:refnum<file>, error out=w118:errorcluster)  [unwired: 4 in, 1 out]
          n52 = Read from Text File(file (use dialog)=w117, error in=w118) -> (refnum out=w116:refnum<file>, text=w124:string, error out=w126:errorcluster)  [unwired: 2 in, 1 out]
          n53 = call <vilib>:"Clear Errors.vi"("error in (no error)"=w126, "specific error code to clear (0: all)"=0) -> ("error out"=w127:errorcluster)  [unwired: 4 in, 1 out]
          n54 = call <vilib>:"Space Constant.vi"() -> ("String"=w110:string)
          n55 = Match Pattern(string=w124, regular expression="정규식 3", offset (0)=34 ("오프셋(0)")) -> (after substring=w113:string)  [unwired: 3 out]
          n56 = Close File(refnum=w116, error in=w127) -> (error out=w108:errorcluster)  [unwired: 1 out]
          n57 = Concatenate Strings(w113, w110, " 일에 lisence 가 등록되었습니다.\n반갑습니다!" ("Message")) -> (w112:string)
          n58 = call "사용자에게 메시지 디스플레이2"("Message"=w112) -> ()  [unwired: 9 in, 2 out]
        }
      }
    }
    frame #1 {
      n59 = disable-structure shown="비활성화" {
        disable-tunnel: w128 -> [w130 _]
        frame Disabled {
          n60 = call "ip address.vi"() -> ("ip address"=w137:string)  [unwired: 11 in]
          "ip address" <- w137
          n61 = call <vilib>:"Space Constant.vi"() -> ("String"=w136:string)
          n62 = call <vilib>:"Space Constant.vi"() -> ("String"=w139:string)
          n63 = Concatenate Strings("serial number ", w139, w130, "의 IP는", w136, w137, w136, "입니다.") -> (w134:string)
          n64 = call "E-메일 보내기"("Message"=w134, "Subject"="ATC appliction customer IP , serial number ") -> ("error out"=w132:errorcluster)  [unwired: 9 in]
          n65 = call <vilib>:"Clear Errors.vi"("error in (no error)"=w132, "specific error code to clear (0: all)"=0) -> ()  [unwired: 4 in, 2 out]
        }
        frame Enabled {
        }
      }
      n66 = for {
        N: 1 -> [_]
        n67 = call "인사말"() -> ()  [unwired: 10 in, 2 out]
      }
    }
    frame #2 {
      n68 = while {
        stop <- FALSE stop-if-true
        n69 = while {
          stop <- FALSE stop-if-true
          n70 = flat-sequence {
            tunnel: [w271] -> w267
            tunnel: "콜사인" -> [w271]
            tunnel: "인사말" -> [w270]
            tunnel: w267 -> [w272]
            tunnel: [w272] -> w266
            tunnel: w266 -> [w273]
            tunnel: [w273] -> w265
            tunnel: w265 -> [w274]
            tunnel: [w274] -> w264
            tunnel: [w275] -> w263
            tunnel: w264 -> [w275]
            tunnel: w263 -> [w276]
            tunnel: [w276] -> w262
            tunnel: [w277] -> w261
            tunnel: w262 -> [w277]
            tunnel: w261 -> [w278]
            tunnel: [w278] -> w260
            tunnel: w260 -> [w279]
            tunnel: [w279] -> w259
            tunnel: w259 -> [w280]
            tunnel: [w280] -> w258
            tunnel: w258 -> [w281]
            tunnel: [w281] -> w257
            tunnel: w257 -> [w282]
            tunnel: [w282] -> w256
            tunnel: w256 -> [w283]
            tunnel: [w283] -> w255
            tunnel: w255 -> [w284]
            frame #0 {
              n71 = local write "인사말2"(w270) -> ()
              n72 = local write "인사말"(w270) -> ()
              n73 = local write "인사말 2"(w270) -> ()
              n74 = local write "인사4"(w270) -> ()
              n75 = local write "인사5"(w270) -> ()
              n76 = local write "인사3"(w270) -> ()
              n77 = local write "콜사인3"(w271) -> ()
              n78 = local write "콜사인2"(w271) -> ()
              n79 = local write "콜사인4"(w271) -> ()
              n80 = local write "콜사인"(w271) -> ()
            }
            frame #1 {
              n81 = local write "콜사인5"(w272) -> ()
              n82 = local write "콜사인6"(w272) -> ()
              n83 = local write "콜사인7"(w272) -> ()
              n84 = local write "콜사인8"(w272) -> ()
            }
            frame #2 {
              n85 = local write "콜사인10"(w273) -> ()
              n86 = local write "콜사인11"(w273) -> ()
              n87 = local write "콜사인9"(w273) -> ()
              n88 = local write "콜사인12"(w273) -> ()
              n89 = local write "콜사인13"(w273) -> ()
              n90 = local write "콜사인14"(w273) -> ()
            }
            frame #3 {
              n91 = local write "콜사인15"(w274) -> ()
              n92 = local write "콜사인16"(w274) -> ()
              n93 = local write "콜사인17"(w274) -> ()
              n94 = local write "콜사인18"(w274) -> ()
              n95 = local write "콜사인19"(w274) -> ()
              n96 = local write "콜사인20"(w274) -> ()
            }
            frame #4 {
              n97 = local write "콜사인21"(w275) -> ()
              n98 = local write "콜사인22"(w275) -> ()
              n99 = local write "콜사인23"(w275) -> ()
              n100 = local write "콜사인24"(w275) -> ()
              n101 = local write "콜사인25"(w275) -> ()
              n102 = local write "콜사인26"(w275) -> ()
            }
            frame #5 {
              n103 = local write "콜사인28"(w276) -> ()
              n104 = local write "콜사인29"(w276) -> ()
              n105 = local write "콜사인30"(w276) -> ()
              n106 = local write "콜사인31"(w276) -> ()
              n107 = local write "콜사인32"(w276) -> ()
            }
            frame #6 {
              n108 = local write "콜사인34 2"(w277) -> ()
              n109 = local write "콜사인33"(w277) -> ()
              n110 = local write "콜사인34"(w277) -> ()
              n111 = local write "콜사인53"(w277) -> ()
              n112 = local write "콜사인54"(w277) -> ()
              n113 = local write "콜사인55"(w277) -> ()
              n114 = local write "콜사인56"(w277) -> ()
            }
            frame #7 {
              n115 = local write "콜사인57"(w278) -> ()
              n116 = local write "콜사인58"(w278) -> ()
              n117 = local write "콜사인59"(w278) -> ()
              n118 = local write "콜사인35"(w278) -> ()
              n119 = local write "콜사인36"(w278) -> ()
              n120 = local write "콜사인37"(w278) -> ()
            }
            frame #8 {
              n121 = local write "콜사인39 2"(w279) -> ()
              n122 = local write "콜사인38"(w279) -> ()
              n123 = local write "콜사인39"(w279) -> ()
              n124 = local write "콜사인40"(w279) -> ()
              n125 = local write "콜사인41"(w279) -> ()
            }
            frame #9 {
              n126 = local write "콜사인38 2"(w280) -> ()
              n127 = local write "콜사인46"(w280) -> ()
              n128 = local write "콜사인47"(w280) -> ()
              n129 = local write "콜사인48"(w280) -> ()
              n130 = local write "콜사인49"(w280) -> ()
              n131 = local write "콜사인50"(w280) -> ()
              n132 = local write "콜사인51"(w280) -> ()
            }
            frame #10 {
              n133 = local write "콜사인60"(w281) -> ()
              n134 = local write "콜사인61"(w281) -> ()
              n135 = local write "콜사인62"(w281) -> ()
              n136 = local write "콜사인63"(w281) -> ()
              n137 = local write "콜사인64"(w281) -> ()
            }
            frame #11 {
              n138 = local write "콜사인65"(w282) -> ()
              n139 = local write "콜사인66"(w282) -> ()
              n140 = local write "콜사인67"(w282) -> ()
              n141 = local write "콜사인68"(w282) -> ()
            }
            frame #12 {
              n142 = local write "콜사인69"(w283) -> ()
              n143 = local write "콜사인69"(w283) -> ()
              n144 = local write "콜사인70"(w283) -> ()
            }
            frame #13 {
              n145 = local write "콜사인72"(w284) -> ()
              n146 = local write "콜사인71"(w284) -> ()
            }
          }
          n147 = flat-sequence {
            tunnel: "L활주로" -> [w287]
            tunnel: [w287] -> w269
            tunnel: w269 -> [w288]
            frame #0 {
              n148 = local write "L활주로3"(w287) -> ()
              n149 = local write "L활주로6"(w287) -> ()
              n150 = local write "L활주로"(w287) -> ()
              n151 = local write "L활주로"(w287) -> ()
              n152 = local write "L활주로"(w287) -> ()
              n153 = local write "L활주로"(w287) -> ()
            }
            frame #1 {
              n154 = local write "L활주로7"(w288) -> ()
              n155 = local write "L활주로"(w288) -> ()
              n156 = local write "L활주로"(w288) -> ()
              n157 = local write "L활주로"(w288) -> ()
            }
          }
          n158 = flat-sequence {
            tunnel: [w285] -> w268
            tunnel: "활주로1" -> [w285]
            tunnel: w268 -> [w286]
            frame #0 {
              n159 = local write "활주로1"(w285) -> ()
              n160 = local write "활주로2"(w285) -> ()
              n161 = local write "활주로3"(w285) -> ()
              n162 = local write "활주로4"(w285) -> ()
              n163 = local write "활주로5"(w285) -> ()
              n164 = local write "활주로6"(w285) -> ()
              n165 = local write "활주로7"(w285) -> ()
            }
            frame #1 {
              n166 = local write "활주로10"(w286) -> ()
              n167 = local write "활주로12"(w286) -> ()
              n168 = local write "활주로13"(w286) -> ()
              n169 = local write "활주로14"(w286) -> ()
              n170 = local write "활주로15"(w286) -> ()
              n171 = local write "활주로8"(w286) -> ()
              n172 = local write "활주로9"(w286) -> ()
            }
          }
          n173 = Wait (ms)(milliseconds to wait=u32 800 ("대기 시간(ms)")) -> ()  [unwired: 1 out]
        }
        n174 = while {
          stop <- FALSE stop-if-true
          # "출발공항의 바람"
          # "도착공항의 바람정보"
          n175 = local write "제한고도2"("제한고도") -> ()
          n176 = local write "T관제기관2"("T관제기관") -> ()
          n177 = local write "ILS2"("ILS") -> ()
          n178 = local write "관제기관3"("T관제기관") -> ()
          n179 = local write "C관제기관2"("C관제기관") -> ()
          n180 = local write "T관제기관3"("T관제기관") -> ()
          n181 = local write "T관제기관"("T관제기관") -> ()
          n182 = local write "T관제기관"("T관제기관") -> ()
          n183 = local write "C관제기관"("C관제기관") -> ()
          n184 = local write "접속주파수2"("접속주파수") -> ()
          n185 = local write "ILS"("ILS") -> ()
          n186 = local write "제한고도"("제한고도") -> ()
          n187 = local write "관제기관"("T관제기관") -> ()
          n188 = local write "관제기관"("T관제기관") -> ()
          n189 = local write "관제기관"("T관제기관") -> ()
          n190 = local write "접속주파수"("접속주파수") -> ()
          n191 = local write "방향 2"("방향") -> ()
          n192 = local write "유도로 2"("유도로 2") -> ()
          n193 = local write "유도로"("유도로 2") -> ()
          n194 = local write "T관제기관4"("T관제기관") -> ()
          n195 = local write "방향"("방향") -> ()
          n196 = local write "고도"("고도") -> ()
          n197 = local write "고도"("고도") -> ()
          n198 = local write "스콱번호"("스콱번호") -> ()
          n199 = local write "스콱번호2"("스콱번호") -> ()
          n200 = local write "T접속주파수2"("T접속주파수") -> ()
          n201 = local write "T접속주파수"("T접속주파수") -> ()
          n202 = local write "허가고도7 3"("허가고도 2") -> ()
          n203 = local write "허가고도7 2"("허가고도 2") -> ()
          n204 = local write "허가고도 2"("허가고도 2") -> ()
          n205 = local write "G관제기관3"("G관제기관") -> ()
          n206 = local write "G관제기관4"("G관제기관") -> ()
          n207 = local write "G관제기관2"("G관제기관") -> ()
          n208 = local write "G관제기관"("G관제기관") -> ()
          n209 = local write "현재기압"("현재기압") -> ()
          n210 = local write "현재기압"("현재기압") -> ()
          n211 = local write "고도"("고도") -> ()
          n212 = local write "고도"("고도") -> ()
          n213 = local write "THEN2"("THEN") -> ()
          n214 = local write "G접속주파수2"("G접속주파수") -> ()
          n215 = local write "THEN"("THEN") -> ()
          n216 = local write "G접속주파수"("G접속주파수") -> ()
          n217 = local write "지점"("지점") -> ()
          n218 = local write "지점 2"("지점") -> ()
          n219 = local write "D관제기관2"("D관제기관") -> ()
          n220 = local write "D관제기관3"("D관제기관") -> ()
          n221 = local write "D관제기관4"("D관제기관") -> ()
          n222 = local write "D관제기관5"("D관제기관") -> ()
          n223 = local write "D관제기관6"("D관제기관") -> ()
          n224 = local write "D관제기관"("D관제기관") -> ()
          n225 = local write "바람방향"("바람방향") -> ()
          n226 = local write "D접속주파수2"("D접속주파수") -> ()
          n227 = local write "D접속주파수"("D접속주파수") -> ()
          n228 = local write "T접속주파수"("T접속주파수") -> ()
          n229 = local write "T접속주파수"("T접속주파수") -> ()
          n230 = local write "A접속주파수2"("A접속주파수") -> ()
          n231 = local write "A접속주파수"("A접속주파수") -> ()
          n232 = local write "풍속"("풍속") -> ()
          n233 = local write "도착공항2"("도착공항") -> ()
          n234 = local write "도착공항3"("도착공항") -> ()
          n235 = local write "도착공항4"("도착공항") -> ()
          n236 = local write "도착공항5"("도착공항") -> ()
          n237 = local write "도착공항"("도착공항") -> ()
          n238 = local write "G접속주파수"("G접속주파수") -> ()
          n239 = local write "G접속주파수"("G접속주파수") -> ()
          n240 = local write "비행고도2"("비행고도") -> ()
          n241 = local write "비행고도3"("비행고도") -> ()
          n242 = local write "비행고도"("비행고도") -> ()
          n243 = local write "A관제기관2"("A관제기관") -> ()
          n244 = local write "A관제기관3"("A관제기관") -> ()
          n245 = local write "A관제기관5"("A관제기관") -> ()
          n246 = local write "A관제기관4"("A관제기관") -> ()
          n247 = local write "A관제기관"("A관제기관") -> ()
          n248 = local write "게이트번호2"("게이트번호") -> ()
          n249 = local write "게이트번호"("게이트번호") -> ()
          n250 = local write "SID&RadarVector. 2"("SID&RadarVector") -> ()
          n251 = local write "SID&RadarVector. 3"("SID&RadarVector") -> ()
          n252 = local write "SID&RadarVector"("SID&RadarVector") -> ()
          n253 = local write "현재기압2"("현재기압") -> ()
          n254 = local write "현재기압"("현재기압") -> ()
          n255 = Wait (ms)(milliseconds to wait=u32 800 ("대기 시간(ms)")) -> ()  [unwired: 1 out]
        }
        n256 = Wait (ms)(milliseconds to wait=u32 0 ("대기 시간(ms)")) -> ()  [unwired: 1 out]
        n257 = while {
          stop <- FALSE stop-if-true
          n258 = Wait (ms)(milliseconds to wait=u32 800 ("대기 시간(ms)")) -> ()  [unwired: 1 out]
          n259 = event shown="[0] \"정보1\": 마우스 커서 들어옴" {
            selector: _ -> [_ _]
            dyn-events: _ -> [_ _]
            timeout: 100 -> [_ _]
            event "정보1": Mouse Enter {
              n260 = event-data() -> ()  [unwired: 1 in, 4 out]
              n261 = call "정보"() -> ()  [unwired: 10 in, 2 out]
            }
            event Timeout {
              n262 = event-data() -> ()  [unwired: 1 in, 3 out]
            }
          }
        }
        n263 = while {
          stop <- FALSE stop-if-true
          n264 = event shown="[1] \"피드백\": 마우스 다운" {
            selector: _ -> [_ _ _]
            dyn-events: _ -> [_ _ _]
            timeout: 10 -> [_ _ _]
            event "도움말": Mouse Up {
              w154 = 128  # call and forget
              n265 = event-data() -> ()  [unwired: 1 in, 8 out]
              n266 = vi-ref "popup.vi"() -> (w147:refnum<vi>)
              n267 = property class="VI"(reference=w147) -> (error out=w148:errorcluster, "Path"=w149:path)  [unwired: 1 in, 1 out]
              n268 = Open VI Reference(type specifier VI Refnum (for type only)=refnum<vi> refnum, vi path=w149, options=w154, error in (no error)=w148) -> (vi reference=w146:refnum<vi>, error out=w152:errorcluster)  [unwired: 2 in]
              n269 = call-by-ref "Start Asynchronous Call"(reference=w146, error in=w152) -> (reference out=w145:refnum<vi>, error out=w151:errorcluster)  [unwired: 12 in]
              n270 = Close Reference(reference=w145, error in (no error)=w151) -> (error out=w150:errorcluster)
              n271 = call <vilib>:"Simple Error Handler.vi"("error in (no error)"=w150) -> ()  [unwired: 4 in, 5 out]
            }
            event "피드백": Mouse Down {
              w164 = 128  # call and forget
              n272 = event-data() -> ()  [unwired: 1 in, 8 out]
              n273 = vi-ref "feedback.vi"() -> (w157:refnum<vi>)
              n274 = property class="VI"(reference=w157) -> (error out=w158:errorcluster, "Path"=w159:path)  [unwired: 1 in, 1 out]
              n275 = Open VI Reference(type specifier VI Refnum (for type only)=refnum<vi> refnum, vi path=w159, options=w164, error in (no error)=w158) -> (vi reference=w156:refnum<vi>, error out=w162:errorcluster)  [unwired: 2 in]
              n276 = call-by-ref "Start Asynchronous Call"(reference=w156, error in=w162) -> (reference out=w155:refnum<vi>, error out=w161:errorcluster)  [unwired: 12 in]
              n277 = Close Reference(reference=w155, error in (no error)=w161) -> (error out=w160:errorcluster)
              n278 = call <vilib>:"Simple Error Handler.vi"("error in (no error)"=w160) -> ()  [unwired: 4 in, 5 out]
            }
            event Timeout {
              n279 = event-data() -> ()  [unwired: 1 in, 3 out]
            }
          }
        }
        n280 = while {
          stop <- FALSE stop-if-true
          n281 = local write "G관제기관"("G관제기관") -> ()
          n282 = local write "관제기관3 2"("G관제기관") -> ()
          n283 = local write "관제기관2"("G관제기관") -> ()
          n284 = local write "관제기관"("G관제기관") -> ()
          n285 = local write "관제기관"("G관제기관") -> ()
          n286 = local write "관제기관4"("G관제기관") -> ()
          n287 = case shown="참" "?" {
            frame False {
            }
            frame True {
              w312 = T3 2 items=["사용자 홈"=0, "사용자 데스크탑"=1, "사용자 문서"=2, "사용자 어플리케이션 데이터"=3, "사용자 환경"=4, "사용자 임시"=5, "퍼블릭 문서"=6, "퍼블릭 어플리케이션 데이터"=7, "퍼블릭 환경"=8, "퍼블릭 캐시"=13, "시스템 코어 라이브러리"=9, "시스템 설치된 라이브러리"=10, "어플리케이션 파일"=11, "부팅 볼륨 루트"=12] ("system directory type")
              n288 = call <vilib>:"Get System Directory.vi"("create directory if not found? (F)"=TRUE, "system directory type"=w312) -> ("system directory"=w314:path)  [unwired: 9 in]
              n289 = Build Path(base path=w314, name or relative path="ATC app output.txt" ("이름 또는 상대 경로")) -> (appended path=w311:path)
              n290 = Open/Create/Replace File(file path (use dialog)=w311) -> (refnum out=w315:refnum<file>, error out=w316:errorcluster)  [unwired: 5 in, 1 out]
              n291 = Read from Text File(file (use dialog)=w315, error in=w316) -> (refnum out=w317:refnum<file>, text=w323:string, error out=w318:errorcluster)  [unwired: 2 in, 1 out]
              n292 = One Button Dialog(message="문서를 불러왔습니다." ("메시지")) -> ()  [unwired: 1 in, 1 out]
              n293 = Match Pattern "Clearance Delivery~Ground"(string=w323, regular expression="Clearance Delivery" ("정규식")) -> (after substring=w320:string)  [unwired: 1 in, 3 out]
              n294 = Close File(refnum=w317, error in=w318) -> ()  [unwired: 2 out]
              n295 = Match Pattern "Clearance Delivery~Ground"(string=w320, regular expression="Ground" ("정규식")) -> (before substring=w325:string, after substring=w324:string)  [unwired: 1 in, 2 out]
              n296 = call <vilib>:"Trim Whitespace.vi"("string"=w325) -> ("trimmed string"=w309:string)  [unwired: 1 in]
              n297 = Match Pattern "Tower(Departure) ~Departure"(string=w324, regular expression="Tower(Departure)" ("정규식")) -> (before substring=w326:string, after substring=w329:string)  [unwired: 1 in, 2 out]
              n298 = local write "메모"(w309) -> ()
              n299 = call <vilib>:"Trim Whitespace.vi"("string"=w326) -> ("trimmed string"=w308:string)  [unwired: 1 in]
              n300 = Match Pattern "Tower(Departure) ~Departure"(string=w329, regular expression="Departure" ("정규식")) -> (before substring=w328:string, after substring=w335:string)  [unwired: 1 in, 2 out]
              n301 = local write "메모2"(w308) -> ()
              n302 = call <vilib>:"Trim Whitespace.vi"("string"=w328) -> ("trimmed string"=w307:string)  [unwired: 1 in]
              n303 = Match Pattern "control~Approach"(string=w335, regular expression="control" ("정규식")) -> (before substring=w333:string, after substring=w331:string)  [unwired: 1 in, 2 out]
              n304 = local write "메모3"(w307) -> ()
              n305 = call <vilib>:"Trim Whitespace.vi"("string"=w333) -> ("trimmed string"=w306:string)  [unwired: 1 in]
              n306 = Match Pattern "control~Approach"(string=w331, regular expression="Approach" ("정규식")) -> (before substring=w334:string, after substring=w303:string)  [unwired: 1 in, 2 out]
              n307 = Match Pattern "Tower(Arrival)~Ground(Arrival)"(string=w303, regular expression="Tower(Arrival)" ("정규식")) -> (before substring=w301:string, after substring=w299:string)  [unwired: 1 in, 2 out]
              n308 = local write "메모 4"(w306) -> ()
              n309 = call <vilib>:"Trim Whitespace.vi"("string"=w334) -> ("trimmed string"=w305:string)  [unwired: 1 in]
              n310 = Match Pattern "Tower(Arrival)~Ground(Arrival)"(string=w299, regular expression="Ground(Arrival)" ("정규식")) -> (before substring=w298:string, after substring=w297:string)  [unwired: 1 in, 2 out]
              n311 = local write "메모6"(w301) -> ()
              n312 = local write "메모5"(w305) -> ()
              n313 = local write "메모7"(w298) -> ()
              n314 = local write "메모8"(w297) -> ()
            }
          }
          n315 = local write "A관제기관5"("G관제기관") -> ()
          n316 = local write "A관제기관3"("G관제기관") -> ()
          n317 = local write "A관제기관4"("G관제기관") -> ()
          n318 = local write "출발공항2"("출발공항") -> ()
          n319 = local write "출발공항"("출발공항") -> ()
          n320 = local write "C활주로3"("C활주로") -> ()
          n321 = local write "C활주로2"("C활주로") -> ()
          n322 = local write "C활주로"("C활주로") -> ()
          n323 = Wait (ms)(milliseconds to wait=u32 800 ("대기 시간(ms)")) -> ()  [unwired: 1 out]
          n324 = local write "허가고도6 3"("허가고도") -> ()
          n325 = local write "허가고도6 2"("허가고도") -> ()
          n326 = local write "허가고도4"("허가고도") -> ()
          n327 = local write "허가고도5"("허가고도") -> ()
          n328 = local write "허가고도6"("허가고도") -> ()
          n329 = local write "허가고도7"("허가고도") -> ()
          n330 = local write "허가고도"("허가고도") -> ()
          n331 = case shown="참" "?" {
            frame False {
            }
            frame True {
              w339 = "\r"
              w347 = "\r"
              w350 = "\r"
              w355 = "\r"
              w364 = T3 2 items=["사용자 홈"=0, "사용자 데스크탑"=1, "사용자 문서"=2, "사용자 어플리케이션 데이터"=3, "사용자 환경"=4, "사용자 임시"=5, "퍼블릭 문서"=6, "퍼블릭 어플리케이션 데이터"=7, "퍼블릭 환경"=8, "퍼블릭 캐시"=13, "시스템 코어 라이브러리"=9, "시스템 설치된 라이브러리"=10, "어플리케이션 파일"=11, "부팅 볼륨 루트"=12] ("system directory type")
              n332 = call <vilib>:"Get System Directory.vi"("create directory if not found? (F)"=TRUE, "system directory type"=w364) -> ("system directory"=w369:path)  [unwired: 9 in]
              n333 = Build Path(base path=w369, name or relative path="ATC app output.txt" ("이름 또는 상대 경로")) -> (appended path=w367:path)
              n334 = One Button Dialog(message="문서 폴더에 저장되었습니다." ("메시지")) -> ()  [unwired: 1 in, 1 out]
              n335 = Concatenate Strings("Clearance Delivery", "\r", "메모", "\r", "Ground", "\r", "메모2", w355, "Tower(Departure)", w355, "메모3", "\r", "Departure", w350, "메모 4", w350, "control", w347, "메모5", w347, "Approach", w347, "메모6", w339, "Tower(Arrival)", w339, "메모7", w339, "Ground(Arrival)", "\r", "메모8") -> (w346:string)
              n336 = Write to Text File(file (use dialog)=w367, text=w346) -> (refnum out=w366:refnum<file>, error out=w365:errorcluster)  [unwired: 2 in, 1 out]
              n337 = Close File(refnum=w366, error in=w365) -> ()  [unwired: 2 out]
            }
          }
        }
        n338 = while {
          stop <- FALSE stop-if-true
          n339 = event shown="[0] 키 다운" {
            selector: _ -> [_ _]
            dyn-events: _ -> [_ _]
            timeout: 0 -> [_ _]
            event Key Down {
              n340 = event-data() -> ("Char"=w169:i16)  [unwired: 1 in, 9 out]
              n341 = Equal?(x=w169, y=i16 43) -> (x = y?=w170:bool)
              n342 = case shown="참" w170 {
                frame False {
                }
                frame True {
                  w175 = T3 2 items=["사용자 홈"=0, "사용자 데스크탑"=1, "사용자 문서"=2, "사용자 어플리케이션 데이터"=3, "사용자 환경"=4, "사용자 임시"=5, "퍼블릭 문서"=6, "퍼블릭 어플리케이션 데이터"=7, "퍼블릭 환경"=8, "퍼블릭 캐시"=13, "시스템 코어 라이브러리"=9, "시스템 설치된 라이브러리"=10, "어플리케이션 파일"=11, "부팅 볼륨 루트"=12] ("system directory type")
                  n343 = call <vilib>:"Get System Directory.vi"("create directory if not found? (F)"=TRUE, "system directory type"=w175) -> ("system directory"=w174:path)  [unwired: 9 in]
                  n344 = Build Path(base path=w174, name or relative path="ATC app output.txt" ("이름 또는 상대 경로")) -> (appended path=w198:path)
                  n345 = Open/Create/Replace File(file path (use dialog)=w198) -> (refnum out=w197:refnum<file>, error out=w196:errorcluster)  [unwired: 5 in, 1 out]
                  n346 = Read from Text File(file (use dialog)=w197, error in=w196) -> (refnum out=w195:refnum<file>, text=w189:string, error out=w194:errorcluster)  [unwired: 2 in, 1 out]
                  n347 = Match Pattern "Clearance Delivery~Ground"(string=w189, regular expression="Clearance Delivery" ("정규식")) -> (after substring=w192:string)  [unwired: 1 in, 3 out]
                  n348 = Close File(refnum=w195, error in=w194) -> ()  [unwired: 2 out]
                  n349 = Match Pattern "Clearance Delivery~Ground"(string=w192, regular expression="Ground" ("정규식")) -> (before substring=w187:string, after substring=w188:string)  [unwired: 1 in, 2 out]
                  n350 = One Button Dialog(message="문서를 불러왔습니다." ("메시지")) -> ()  [unwired: 1 in, 1 out]
                  n351 = call <vilib>:"Trim Whitespace.vi"("string"=w187) -> ("trimmed string"=w199:string)  [unwired: 1 in]
                  n352 = Match Pattern "Tower(Departure) ~Departure"(string=w188, regular expression="Tower(Departure)" ("정규식")) -> (before substring=w186:string, after substring=w183:string)  [unwired: 1 in, 2 out]
                  n353 = local write "메모"(w199) -> ()
                  n354 = call <vilib>:"Trim Whitespace.vi"("string"=w186) -> ("trimmed string"=w200:string)  [unwired: 1 in]
                  n355 = Match Pattern "Tower(Departure) ~Departure"(string=w183, regular expression="Departure" ("정규식")) -> (before substring=w184:string, after substring=w177:string)  [unwired: 1 in, 2 out]
                  n356 = local write "메모2"(w200) -> ()
                  n357 = call <vilib>:"Trim Whitespace.vi"("string"=w184) -> ("trimmed string"=w201:string)  [unwired: 1 in]
                  n358 = Match Pattern "control~Approach"(string=w177, regular expression="control" ("정규식")) -> (before substring=w179:string, after substring=w181:string)  [unwired: 1 in, 2 out]
                  n359 = local write "메모3"(w201) -> ()
                  n360 = call <vilib>:"Trim Whitespace.vi"("string"=w179) -> ("trimmed string"=w202:string)  [unwired: 1 in]
                  n361 = Match Pattern "control~Approach"(string=w181, regular expression="Approach" ("정규식")) -> (before substring=w178:string, after substring=w205:string)  [unwired: 1 in, 2 out]
                  n362 = Match Pattern "Tower(Arrival)~Ground(Arrival)"(string=w205, regular expression="Tower(Arrival)" ("정규식")) -> (before substring=w207:string, after substring=w209:string)  [unwired: 1 in, 2 out]
                  n363 = local write "메모 4"(w202) -> ()
                  n364 = call <vilib>:"Trim Whitespace.vi"("string"=w178) -> ("trimmed string"=w203:string)  [unwired: 1 in]
                  n365 = Match Pattern "Tower(Arrival)~Ground(Arrival)"(string=w209, regular expression="Ground(Arrival)" ("정규식")) -> (before substring=w210:string, after substring=w211:string)  [unwired: 1 in, 2 out]
                  n366 = local write "메모6"(w207) -> ()
                  n367 = local write "메모5"(w203) -> ()
                  n368 = local write "메모7"(w210) -> ()
                  n369 = local write "메모8"(w211) -> ()
                }
              }
              n370 = Equal?(x=w169, y=i16 45) -> (x = y?=w172:bool)
              n371 = case shown="참" w172 {
                frame False {
                }
                frame True {
                  w215 = "\r"
                  w228 = "\r"
                  w230 = "\r"
                  w233 = "\r"
                  w240 = T3 2 items=["사용자 홈"=0, "사용자 데스크탑"=1, "사용자 문서"=2, "사용자 어플리케이션 데이터"=3, "사용자 환경"=4, "사용자 임시"=5, "퍼블릭 문서"=6, "퍼블릭 어플리케이션 데이터"=7, "퍼블릭 환경"=8, "퍼블릭 캐시"=13, "시스템 코어 라이브러리"=9, "시스템 설치된 라이브러리"=10, "어플리케이션 파일"=11, "부팅 볼륨 루트"=12] ("system directory type")
                  n372 = local read "메모6"() -> (w218:string)
                  n373 = local read "메모5"() -> (w219:string)
                  n374 = local read "메모 4"() -> (w220:string)
                  n375 = local read "메모7"() -> (w216:string)
                  n376 = local read "메모2"() -> (w222:string)
                  n377 = local read "메모3"() -> (w221:string)
                  n378 = local read "메모"() -> (w223:string)
                  n379 = local read "메모8"() -> (w212:string)
                  n380 = One Button Dialog(message="문서 폴더에 저장되었습니다." ("메시지")) -> ()  [unwired: 1 in, 1 out]
                  n381 = Concatenate Strings("Clearance Delivery", "\r", w223, "\r", "Ground", "\r", w222, w233, "Tower(Departure)", w233, w221, "\r", "Departure", w230, w220, w230, "control", w228, w219, w228, "Approach", w228, w218, w215, "Tower(Arrival)", w215, w216, w215, " Ground(Arrival)", "\r", w212) -> (w227:string)
                  n382 = call <vilib>:"Get System Directory.vi"("create directory if not found? (F)"=TRUE, "system directory type"=w240) -> ("system directory"=w245:path)  [unwired: 9 in]
                  n383 = Build Path(base path=w245, name or relative path="ATC app output.txt" ("이름 또는 상대 경로")) -> (appended path=w243:path)
                  n384 = Write to Text File(file (use dialog)=w243, text=w227) -> (refnum out=w242:refnum<file>, error out=w241:errorcluster)  [unwired: 2 in, 1 out]
                  n385 = Close File(refnum=w242, error in=w241) -> ()  [unwired: 2 out]
                }
              }
            }
            event Timeout {
              n386 = event-data() -> ()  [unwired: 1 in, 3 out]
            }
          }
          n387 = Wait (ms)(milliseconds to wait=u32 800 ("대기 시간(ms)")) -> ()  [unwired: 1 out]
        }
      }
    }
  }
